vi "XSens Msg Size (SubVI).vi"(11 "From Q":string) -> (1 "Data Size":u16, 3 "Index":i16)   [LabVIEW 2019]
doc: "Takes the Xsens hex string data from queue (or Stream Channel) and extracts the data size and outputs new indexing values. Should handle the extended message size (2 byte value), but have not yet tested since all data thus far fits in the standard 1 byte format. \n\nData in should be all bytes after the preamble (FA)\n\n2020 NREL"
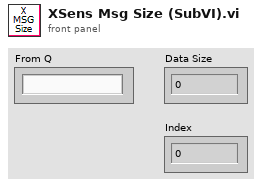
[diagram p1: front panel]
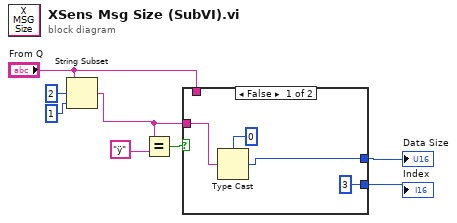
[diagram p0: block diagram]
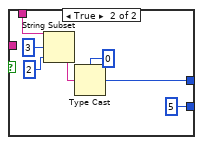
[diagram p2: hidden frame]
diagram:
  n1 = String Subset(string="From Q", offset (0)=2, length (rest)=1 ("length (rest)")) -> (substring=w5:string)
  n2 = Equal?(x=w5, y="ÿ") -> (x = y?=w4:bool)
  n3 = case shown="False" w4 {
    tunnel: w5 -> [w11 _]
    tunnel: [w10 w18] -> w6
    tunnel: "From Q" -> [_ w16]
    tunnel: [i16 3 ("offset (0)") i16 5 ("offset (0)")] -> w8
    frame False {
      n4 = Type Cast(type=u8 0, x=w11) -> (*(type *) &x=w10:u8)
    }
    frame True {
      n5 = String Subset(string=w16, offset (0)=i16 3, length (rest)=2 ("length (rest)")) -> (substring=w15:string)
      n6 = Type Cast(type=u16 0, x=w15) -> (*(type *) &x=w18:u16)
    }
  }
  "Data Size" <- w6
  "Index" <- w8
